vi "Print Roi Array.vi"(11 "Roi Array":T1[](array[typedef])) -> (0 "error out":errorcluster, 3 "String":string)   [LabVIEW 2020, in "Camera.lvlib"]
uses:
  Camera.lvlib
  ROI--cluster.ctl
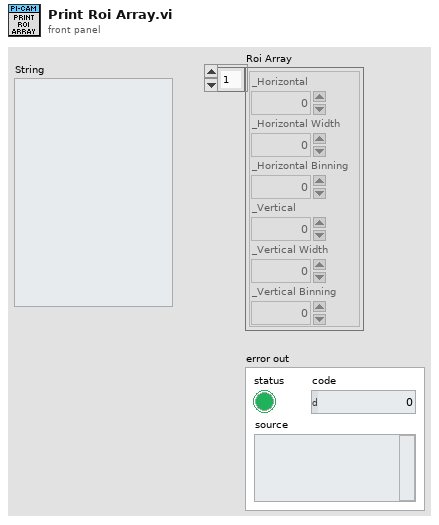
[diagram p1: front panel]
types:
  T1 = typedef "Camera.lvlib/ROI--cluster.ctl" = cluster{"_Horizontal":i32, "_Horizontal Width":i32, "_Horizontal Binning":i32, "_Vertical":i32, "_Vertical Width":i32, "_Vertical Binning":i32}
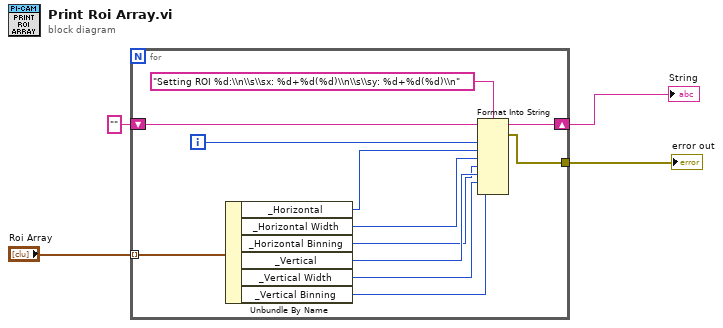
[diagram p0: block diagram]
diagram:
  n1 = for {
    tunnel: [w11] -> w4
    tunnel: "Roi Array" -> [w6] mode=indexing
    shift-right: [w10] -> w3
    shift-left: "" -> [w5]
    i -> [w7]
    n2 = Unbundle By Name(w6) -> ("_Horizontal"=w8:i32, "_Horizontal Width"=w12:i32, "_Horizontal Binning"=w13:i32, "_Vertical"=w14:i32, "_Vertical Width"=w15:i32, "_Vertical Binning"=w16:i32)
    n3 = Format Into String(format string="Setting ROI %d:\\n\\s\\sx: %d+%d(%d)\\n\\s\\sy: %d+%d(%d)\\n", initial string=w5, w7, w8, w12, w13, w14, w15, w16) -> (resulting string=w10:string, error out=w11:errorcluster)  [unwired: 1 in]
  }
  "error out" <- w4
  "String" <- w3
